vi "t-trigger.vi"(2 "S":bool, 3 "T":bool, 4 "R":bool) -> (0 "notQ":bool, 1 "Q":bool)   [LabVIEW 2013]
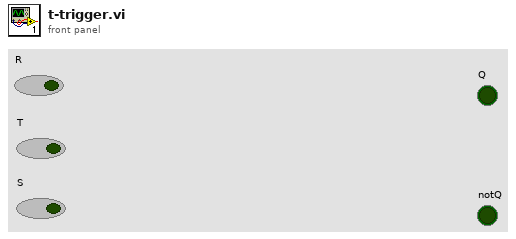
[diagram p1: front panel]
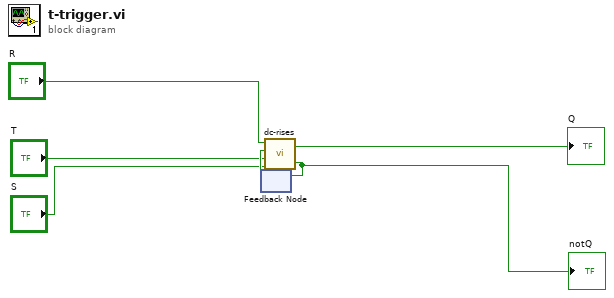
[diagram p0: block diagram]
diagram:
  n1 = feedback #1() -> (w6:bool)  [unwired: 1 in]
  n2 = call "dc-rises.vi"("S"="S", "C"="T", "D"=w6, "R"="R") -> ("notQ"=w3:bool, "Q"=→"Q":bool)
  "notQ" <- w3
  n3 = feedback-in #1(w3) -> ()
